vi "Lidar 오브젝트화.vi"() -> ()   [LabVIEW 2016]
uses:
  <vilib>/Platform/TimedLoop/XDataNode/timing_clust.ctl
  <vilib>/Platform/TimedLoop/XDataNode/nitl_modes.ctl
  <vilib>/Platform/TimedLoop/XDataNode/wakeup.ctl
  <vilib>/imath/engines/lvmath2/RunTimeEngine/Managers/WorkSpace/UID Generator.vi
  <vilib>/imath/engines/lvmath2/RunTimeEngine/IndexRead/NIMS M($,S).vi
  <instcachedir>/0/NIMS M($,S)_3E5749BBB62E49528D4765A77F1F6D98.lvgen/NIMS M($,S)_3E5749BBB62E49528D4765A77F1F6D98_000.vi
  <vilib>/imath/engines/lvmath2/RunTimeEngine/RunTimeType/NIMS_RunTimeType_From StrictType (excl LVString).vi
  <instcachedir>/0/NIMS_RunTimeType_From StrictType (excl LVString)_BBF44FB49F834B71AF7A14CCEDF8BECD.lvgen/NIMS_RunTimeType_From StrictType (excl LVString)_BBF44FB49F834B71AF7A14CCEDF8BECD_000.vi
  <vilib>/imathl/engines/lvmath/Functions/Error Handling/Create Error.vi
  <vilib>/imath/engines/lvmath2/RunTimeEngine/LocalVariableDefStatement/MC_LocalVariableDefStatement_Display.vi
  <vilib>/imath/engines/lvmath2/RunTimeEngine/BuiltInFunctions/deg_to_rad/NIMS_deg_to_rad.vi
  <instcachedir>/0/NIMS_deg_to_rad_4A81D684CE8D4DD79924F5AB74D756E1.lvgen/NIMS_deg_to_rad_4A81D684CE8D4DD79924F5AB74D756E1_002.vi
  <vilib>/imath/engines/lvmath2/RunTimeEngine/ArithmeticOperatorToken/NIMS_ArithmeticOperator_times.vi
  <instcachedir>/0/NIMS_ArithmeticOperator_times_953B34F74CAC448FB707D816A29CC5F0.lvgen/NIMS_ArithmeticOperator_times_953B34F74CAC448FB707D816A29CC5F0_000.vi
  <vilib>/imath/engines/lvmath2/RunTimeEngine/IndexReplace/NIMS M($,S)=V.vi
  <instcachedir>/0/NIMS M($,S)=V_EEA74323A7E5479BB387BE0F93352290.lvgen/NIMS M($,S)=V_EEA74323A7E5479BB387BE0F93352290_001.vi
  <vilib>/imath/engines/lvmath2/RunTimeEngine/ErrorHandling/NIMS_Create Error From Enums.vi
  <vilib>/imath/engines/lvmath2/RunTimeEngine/IndexRead/NIMS M(S,S).vi
  <instcachedir>/0/NIMS M(S,S)_AC51E74150A542F7991B9634C66F3096.lvgen/NIMS M(S,S)_AC51E74150A542F7991B9634C66F3096_000.vi
  <vilib>/imath/engines/lvmath2/RunTimeEngine/BuiltInFunctions/size/NIMS_I32Row=size(GM).vi
  <instcachedir>/0/NIMS_I32Row=size(GM)_10ACDCB9F1F84A7E9F42C91D87611FB5.lvgen/NIMS_I32Row=size(GM)_10ACDCB9F1F84A7E9F42C91D87611FB5_001.vi
  <vilib>/imath/engines/lvmath2/RunTimeEngine/IndexRead/NIMS V(S).vi
  <instcachedir>/0/NIMS V(S)_0488751826AF41519A22953C041130DC.lvgen/NIMS V(S)_0488751826AF41519A22953C041130DC_002.vi
  <vilib>/imath/engines/lvmath2/RunTimeEngine/IndexRead/NIMS M(R2,S).vi
  <instcachedir>/0/NIMS M(R2,S)_56813DCFDD5A484292D2195AF15D2BF5.lvgen/NIMS M(R2,S)_56813DCFDD5A484292D2195AF15D2BF5_000.vi
  <vilib>/imath/engines/lvmath2/RunTimeEngine/ArithmeticOperatorToken/NIMS_ArithmeticOperator_minus.vi
  <instcachedir>/0/NIMS_ArithmeticOperator_minus_E3B65B1D26A44BB184AFDC5B3F458E3D.lvgen/NIMS_ArithmeticOperator_minus_E3B65B1D26A44BB184AFDC5B3F458E3D_003.vi
  <vilib>/imath/engines/lvmath2/RunTimeEngine/ArithmeticOperatorToken/NIMS_ArithmeticOperator_plus.vi
  <instcachedir>/0/NIMS_ArithmeticOperator_plus_0120E0498A0F4B4B9BDCAC2554767A4E.lvgen/NIMS_ArithmeticOperator_plus_0120E0498A0F4B4B9BDCAC2554767A4E_004.vi
  <vilib>/imath/engines/lvmath2/RunTimeEngine/Managers/SymbolTable/Clear UID.vi
  <vilib>/imath/engines/lvmath2/RunTimeEngine/NodeEndStatement/NIMS_NodeEndStatement_Output.vi
  <instcachedir>/0/NIMS_NodeEndStatement_Output_53EC0D466D134D7ABD903AC30B43404B.lvgen/NIMS_NodeEndStatement_Output_53EC0D466D134D7ABD903AC30B43404B_005.vi
  <instcachedir>/0/NIMS_NodeEndStatement_Output_53EC0D466D134D7ABD903AC30B43404B.lvgen/NIMS_NodeEndStatement_Output_53EC0D466D134D7ABD903AC30B43404B_004.vi
  <instcachedir>/0/NIMS_NodeEndStatement_Output_53EC0D466D134D7ABD903AC30B43404B.lvgen/NIMS_NodeEndStatement_Output_53EC0D466D134D7ABD903AC30B43404B_010.vi
  <instcachedir>/0/NIMS_NodeEndStatement_Output_53EC0D466D134D7ABD903AC30B43404B.lvgen/NIMS_NodeEndStatement_Output_53EC0D466D134D7ABD903AC30B43404B_002.vi
  <instcachedir>/0/NIMS_NodeEndStatement_Output_53EC0D466D134D7ABD903AC30B43404B.lvgen/NIMS_NodeEndStatement_Output_53EC0D466D134D7ABD903AC30B43404B_001.vi
  <vilib>/imath/engines/lvmath2/RunTimeEngine/ErrorHandling/NIMS_Finalize Error.vi
  <vilib>/imath/engines/lvmath2/RunTimeEngine/ArithmeticOperatorToken/NIMS_ArithmeticOperator_rightdiv.vi
  <instcachedir>/0/NIMS_ArithmeticOperator_rightdiv_0403F5D95ED04A4080FE3DA43A6A83B7.lvgen/NIMS_ArithmeticOperator_rightdiv_0403F5D95ED04A4080FE3DA43A6A83B7_000.vi
  <vilib>/imath/engines/lvmath2/RunTimeEngine/RowToken/NIMS_RowToken_CV_CV.vi
  <instcachedir>/0/NIMS_RowToken_CV_CV_5546A0B1CA2C4E49826F811B9C073FB0.lvgen/NIMS_RowToken_CV_CV_5546A0B1CA2C4E49826F811B9C073FB0_001.vi
  <vilib>/Platform/TimedLoop/XDataNode/XDataNode.xnode
  <vilib>/Platform/TimedLoop/XDataNode/XDNodeRunTimeDep.lvlib
  <vilib>/imath/engines/lvmath2/RunTimeEngine/Managers/SymbolTable/NIMS_WorkSpace.lvlib
panel:
  out "X":dbl[][](array[numeric])
  out "arraysize":i32[](array[numeric])
  out "row":i32
  out "x1":dbl
  out "y1":dbl
  out "x init":dbl
  out "y init":dbl
  out "오브젝트":cluster{dbl[], dbl[]}(graph)
  in  "오브젝트화 제한 거리":dbl=200.0
  out "x2":dbl
  out "y2":dbl
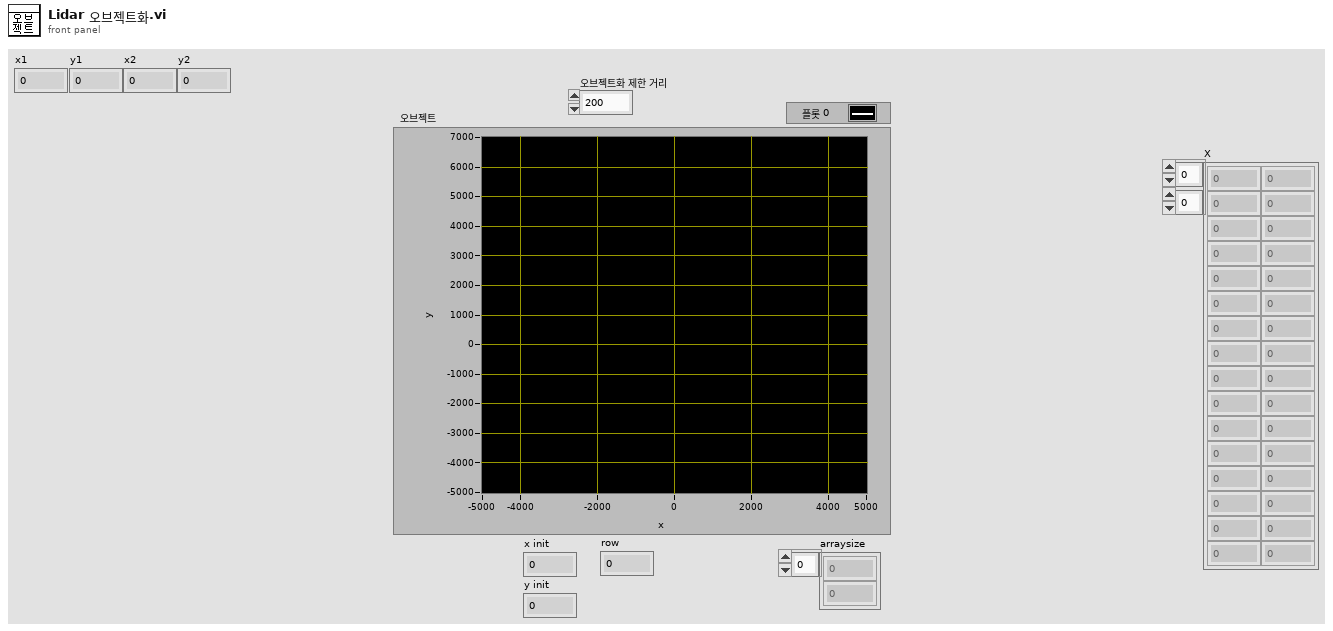
[diagram p1: front panel]
types:
  T1 = typedef "XDNodeRunTimeDep.lvlib/timing_clust.ctl" = cluster{"Expected End [f-1]":u64, "Actual End [f-1]":u64, "Finished Late? [f-1]":bool, "Expected End [i-1]":u64, "Actual End [i-1]":u64, "Finished Late? [i-1]":bool, "Expected Start [i]":u64, "Actual Start [i]":u64, "Expected Start [f]":u64, "Actual Start [f]":u64, "Source Name":string, "Structure Name":string, "Period":i64, "Deadline":i64, "Offset":i64, "Start":i64, "Priority":i32, "Timeout":i32, "Mode":T2, "Wakeup Reason":T3, "Error":errorcluster, "Source Type":string, "Secondary Source Type":string, "Global End Time":u64, "Global Start Time":u64, "Frame Duration":u64, "Iteration Duration":u64, "Assigned CPU":i32, "I/O Scan Engine Mode":u32}
  T2 = typedef "XDNodeRunTimeDep.lvlib/nitl_modes.ctl" = enum32{"No Change", "Process missed periods, maintain original phase", "Discard missed periods, maintain original phase", "Process missed periods, ignore original phase", "Discard missed periods, ignore original phase"}
  T3 = typedef "XDNodeRunTimeDep.lvlib/wakeup.ctl" = enum32{"Normal", "Aborted", "Asynchronous wakeup", "Timing source error", "Timed loop error", "Timeout"}
  T4 = typedef "2차원배열 공유변수.ctl" = dbl[][]
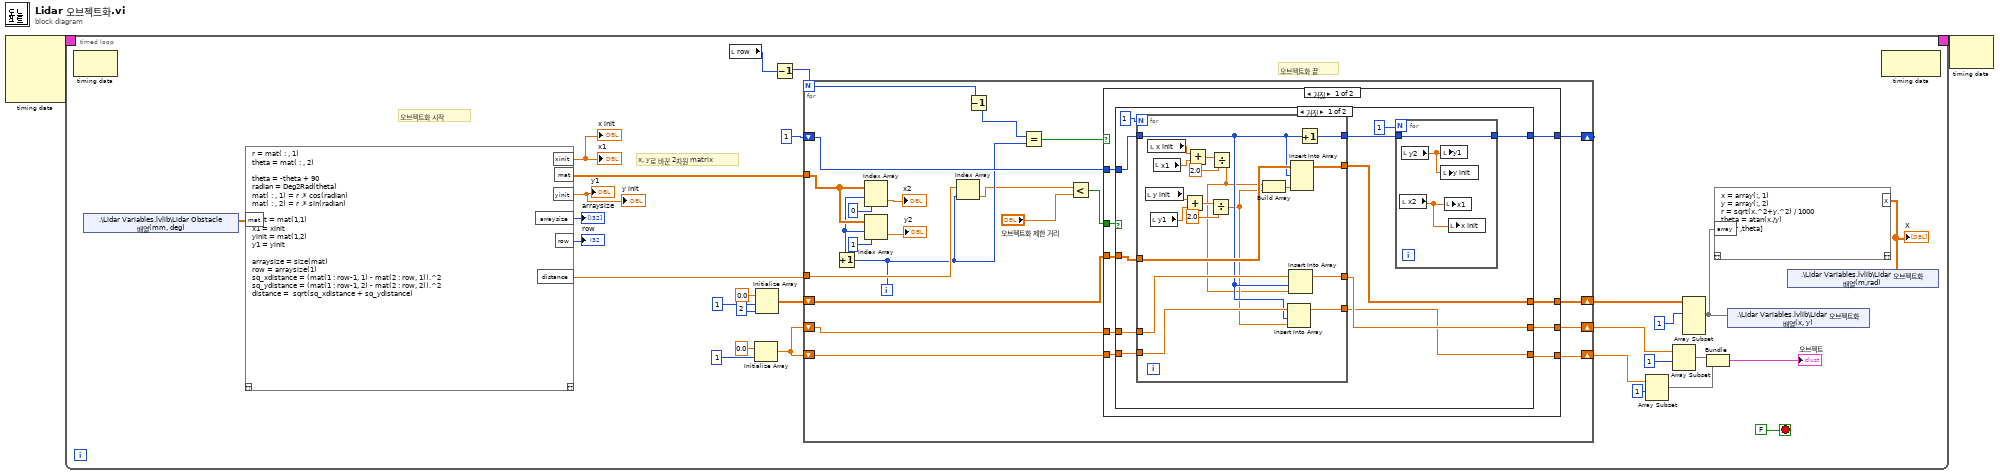
[diagram p0: block diagram]
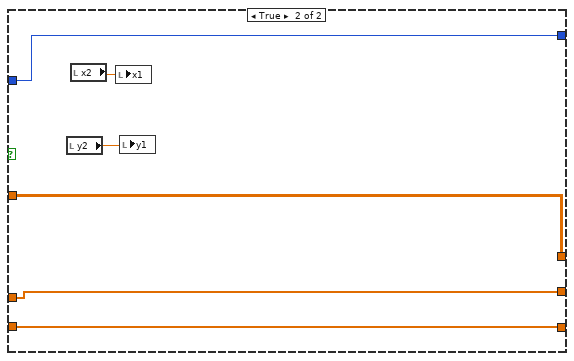
[diagram p2: hidden frame]
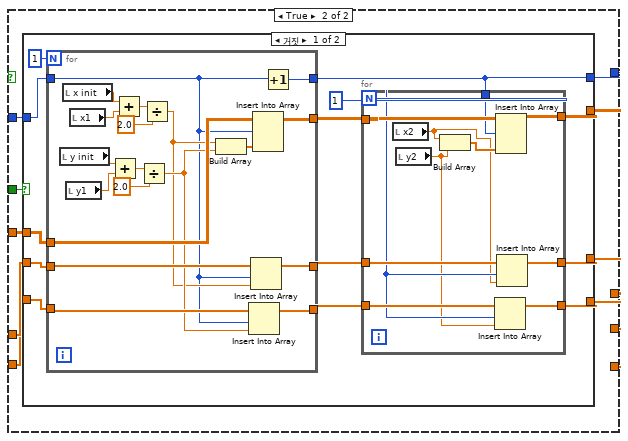
[diagram p3: hidden frame]
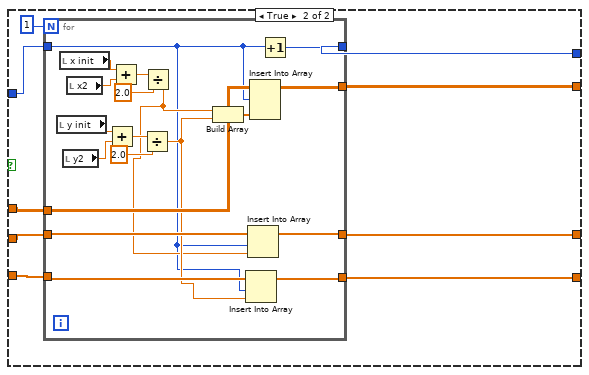
[diagram p4: hidden frame]
diagram:
  n1 = node-c288() -> (w2:T1)  [unwired: 4 in]
  n2 = timed-loop {
    timing: w2 -> [_]
    timing-out: [_] -> w1
    stop <- FALSE stop-if-true
    # "x, y로 바꾼 2차원 matrix"
    # "오브젝트화 끝"
    # "오브젝트화 시작"
    n3 = node-c288() -> ()  [unwired: 1 in, 1 out]
    n4 = shared-variable ".\\Lidar Variables.lvlib\\Lidar Obstacle 배열(mm, deg)"() -> (w5:T4)  [unwired: 1 in, 1 out]
    n5 = mathscript code="r = mat( : , 1)\ntheta = mat( : , 2)\n\ntheta = -theta + 90\nradian = Deg2Rad(theta)\nmat( : , 1) = r .* cos(radian)\nmat( : , 2) = r .* sin(radian)\n\nxinit = mat(1,1)\nx1 = xinit\nyinit = mat(1,2)\ny1 = yinit\n\narraysize = size(mat)\nrow = arraysize(1)\nsq_xdistance = (mat(1 : row-1, 1) - mat(2 : row, 1)).^2\nsq_ydistance = (mat(1 : row-1, 2) - mat(2 : row, 2)).^2\ndistance =  sqrt(sq_xdistance + sq_ydistance)"("mat"=w5) -> ("xinit"=→"x1" →"x init":dbl, "yinit"=→"y1" →"y init":dbl, "mat"=w11:dbl[][], "row"=→"row":i32, "arraysize"=→"arraysize":i32[], "distance"=w8:dbl[])  [unwired: 1 in, 1 out]
    n6 = local read "row"() -> (w7:i32)
    n7 = Initialize Array(0.0 ("원소"), 1 ("차원 크기")) -> (w25:dbl[])
    n8 = Initialize Array(0.0 ("원소"), 1 ("차원 크기"), 2 ("차원 크기")) -> (w15:dbl[][])
    n9 = Decrement(x=w7) -> (x-1=w16:i32)
    n10 = for {
      N: w16 -> [w651]
      tunnel: w11 -> [w644]
      shift-right: [w655] -> _
      shift-left: 1 -> [w656]
      shift-right: [w648] -> w24
      shift-left: w15 -> [w654]
      shift-right: [w647] -> w20
      shift-left: w25 -> [w653]
      shift-right: [w637] -> w6
      shift-left: w25 -> [w652]
      tunnel: w8 -> [w640]
      i -> [w639]
      n11 = Increment(x=w639) -> (x+1=w641:i32)
      n12 = Index Array(array=w644, index (row)=w641, index (col)=0 ("비활성화된 인덱스 (열)")) -> (element=→"x2":dbl)
      n13 = Index Array(array=w644, index (row)=w641, index (col)=1 ("비활성화된 인덱스 (열)")) -> (element=→"y2":dbl)
      n14 = Index Array(array=w640, index=w639) -> (element=w638:dbl)
      n15 = Decrement(x=w651) -> (x-1=w650:i32)
      n16 = Equal?(x=w650, y=w639) -> (x = y?=w649:bool)
      n17 = Less?(x=w638, y="오브젝트화 제한 거리") -> (x < y?=w657:bool)
      n18 = case shown="거짓" w649 {
        tunnel: w657 -> [w667 w710]
        tunnel: w656 -> [w666 w712]
        tunnel: [w665 w711] -> w655
        tunnel: w654 -> [w664 w715]
        tunnel: w653 -> [w663 w714]
        tunnel: w652 -> [w662 w713]
        tunnel: [w660 w709] -> w648
        tunnel: [w661 w708] -> w647
        tunnel: [w659 w707] -> w637
        frame False {
          n19 = case shown="거짓" w667 {
            tunnel: w664 -> [w678 w705]
            tunnel: w666 -> [w677 w706]
            tunnel: [w672 w706] -> w665
            tunnel: [w670 w705] -> w660
            tunnel: w663 -> [w675 w701]
            tunnel: w662 -> [w674 w702]
            tunnel: [w669 w701] -> w661
            tunnel: [w668 w702] -> w659
            frame False {
              n20 = for {
                N: 1 -> [_]
                tunnel: w678 -> [w692]
                tunnel: [w689] -> w670
                tunnel: w675 -> [w688]
                tunnel: w674 -> [w686]
                tunnel: [w687] -> w669
                tunnel: [w685] -> w668
                tunnel: w677 -> [w684]
                tunnel: [w690] -> w673
                n21 = local read "y init"() -> (w693:dbl)
                n22 = local read "x init"() -> (w699:dbl)
                n23 = local read "y1"() -> (w694:dbl)
                n24 = local read "x1"() -> (w700:dbl)
                n25 = Add(x=w693, y=w694) -> (x+y=w695:dbl)
                n26 = Add(x=w699, y=w700) -> (x+y=w698:dbl)
                n27 = Divide(x=w695, y=2.0) -> (x/y=w683:dbl)
                n28 = Divide(x=w698, y=2.0) -> (x/y=w682:dbl)
                n29 = Build Array(w682, w683) -> (w691:dbl[])
                n30 = Insert Into Array(array=w686, index=w684, new element=w683) -> (w685:dbl[])
                n31 = Insert Into Array(array=w688, index=w684, new element=w682) -> (w687:dbl[])
                n32 = Insert Into Array(array=w692, index (row)=w684, new element=w691) -> (w689:dbl[][])  [unwired: 1 in]
                n33 = Increment(x=w684) -> (x+1=w690:i32)
              }
              n34 = for {
                N: 1 -> [_]
                tunnel: w673 -> [w679]
                tunnel: [w679] -> w672
                n35 = local read "x2"() -> (w680:dbl)
                n36 = local read "y2"() -> (w681:dbl)
                n37 = local write "y1"(w681) -> ()
                n38 = local write "y init"(w681) -> ()
                n39 = local write "x1"(w680) -> ()
                n40 = local write "x init"(w680) -> ()
              }
            }
            frame True {
              n41 = local read "y2"() -> (w704:dbl)
              n42 = local read "x2"() -> (w703:dbl)
              n43 = local write "x1"(w703) -> ()
              n44 = local write "y1"(w704) -> ()
            }
          }
        }
        frame True {
          n45 = case shown="거짓" w710 {
            tunnel: w715 -> [w727 w765]
            tunnel: w714 -> [w726 w764]
            tunnel: w713 -> [w725 w763]
            tunnel: [w718 w762] -> w708
            tunnel: [w717 w761] -> w707
            tunnel: w712 -> [w724 w760]
            tunnel: [w719 w759] -> w711
            tunnel: [w722 w758] -> w709
            frame False {
              n46 = for {
                N: 1 -> [_]
                tunnel: w727 -> [w749]
                tunnel: [w746] -> w723
                tunnel: w726 -> [w745]
                tunnel: w725 -> [w743]
                tunnel: [w744] -> w721
                tunnel: [w742] -> w720
                tunnel: w724 -> [w739]
                tunnel: [w747] -> w719
                n47 = local read "y init"() -> (w750:dbl)
                n48 = local read "x init"() -> (w756:dbl)
                n49 = local read "y1"() -> (w751:dbl)
                n50 = local read "x1"() -> (w757:dbl)
                n51 = Add(x=w750, y=w751) -> (x+y=w752:dbl)
                n52 = Add(x=w756, y=w757) -> (x+y=w755:dbl)
                n53 = Divide(x=w752, y=2.0) -> (x/y=w741:dbl)
                n54 = Divide(x=w755, y=2.0) -> (x/y=w740:dbl)
                n55 = Build Array(w740, w741) -> (w748:dbl[])
                n56 = Insert Into Array(array=w743, index=w739, new element=w741) -> (w742:dbl[])
                n57 = Insert Into Array(array=w745, index=w739, new element=w740) -> (w744:dbl[])
                n58 = Insert Into Array(array=w749, index (row)=w739, new element=w748) -> (w746:dbl[][])  [unwired: 1 in]
                n59 = Increment(x=w739) -> (x+1=w747:i32)
              }
              n60 = for {
                N: 1 -> [_]
                tunnel: w723 -> [w738]
                tunnel: [w737] -> w722
                tunnel: w721 -> [w735]
                tunnel: w720 -> [w734]
                tunnel: w719 -> [w733]
                tunnel: [w732] -> w718
                tunnel: [w731] -> w717
                n61 = local read "x2"() -> (w730:dbl)
                n62 = local read "y2"() -> (w729:dbl)
                n63 = Build Array(w730, w729) -> (w736:dbl[])
                n64 = Insert Into Array(array=w734, index=w733, new element=w729) -> (w731:dbl[])
                n65 = Insert Into Array(array=w738, index (row)=w733, new element=w736) -> (w737:dbl[][])  [unwired: 1 in]
                n66 = Insert Into Array(array=w735, index=w733, new element=w730) -> (w732:dbl[])
              }
            }
            frame True {
              n67 = for {
                N: 1 -> [_]
                tunnel: w765 -> [w777]
                tunnel: [w774] -> w758
                tunnel: w764 -> [w773]
                tunnel: w763 -> [w771]
                tunnel: [w772] -> w762
                tunnel: [w770] -> w761
                tunnel: w760 -> [w767]
                tunnel: [w775] -> w759
                n68 = local read "y init"() -> (w778:dbl)
                n69 = local read "x init"() -> (w784:dbl)
                n70 = local read "y2"() -> (w779:dbl)
                n71 = local read "x2"() -> (w785:dbl)
                n72 = Add(x=w778, y=w779) -> (x+y=w780:dbl)
                n73 = Add(x=w784, y=w785) -> (x+y=w783:dbl)
                n74 = Divide(x=w780, y=2.0) -> (x/y=w769:dbl)
                n75 = Divide(x=w783, y=2.0) -> (x/y=w768:dbl)
                n76 = Build Array(w768, w769) -> (w776:dbl[])
                n77 = Insert Into Array(array=w771, index=w767, new element=w769) -> (w770:dbl[])
                n78 = Insert Into Array(array=w773, index=w767, new element=w768) -> (w772:dbl[])
                n79 = Insert Into Array(array=w777, index (row)=w767, new element=w776) -> (w774:dbl[][])  [unwired: 1 in]
                n80 = Increment(x=w767) -> (x+1=w775:i32)
              }
            }
          }
        }
      }
    }
    n81 = Array Subset(array=w6, index=1 ("인덱스")) -> (w18:dbl[])  [unwired: 1 in]
    n82 = Array Subset(array=w20, index=1 ("인덱스")) -> (w19:dbl[])  [unwired: 1 in]
    n83 = Array Subset(array=w24, index (row)=1 ("인덱스")) -> (w3:dbl[][])  [unwired: 3 in]
    n84 = Bundle(w19, w18) -> (→"오브젝트":cluster{dbl[], dbl[]})  [unwired: 1 in]
    n85 = mathscript code="x = array(:, 1)\ny = array(:, 2)\nr = sqrt(x.^2+y.^2) / 1000\ntheta = atan(x./y)\nX=[r ,theta]"("array"=w3) -> ("X"=w4:dbl[][])  [unwired: 1 in, 1 out]
    "X" <- w4
    n86 = shared-variable ".\\Lidar Variables.lvlib\\Lidar 오브젝트화 배열(x, y)"(w3) -> ()  [unwired: 1 in, 1 out]
    n87 = shared-variable ".\\Lidar Variables.lvlib\\Lidar 오브젝트화 배열(m,rad)"(w4) -> ()  [unwired: 1 in, 1 out]
    n88 = node-c288() -> ()  [unwired: 1 in, 1 out]
  }
  n89 = node-c288(w1) -> ()  [unwired: 1 out]
